vi "xlsx to Cluster.vi"(7 "Excel._SheetName":string="Sheet1", 8 "Error (in)":errorcluster, 11 "file path (dialog if empty)":path) -> (0 "Error (out)":errorcluster, 3 "Parameter Array":T1[](array[typedef]))   [LabVIEW 2020]
uses:
  Controls/Database_Array.ctl
  Controls/Encoding.ctl
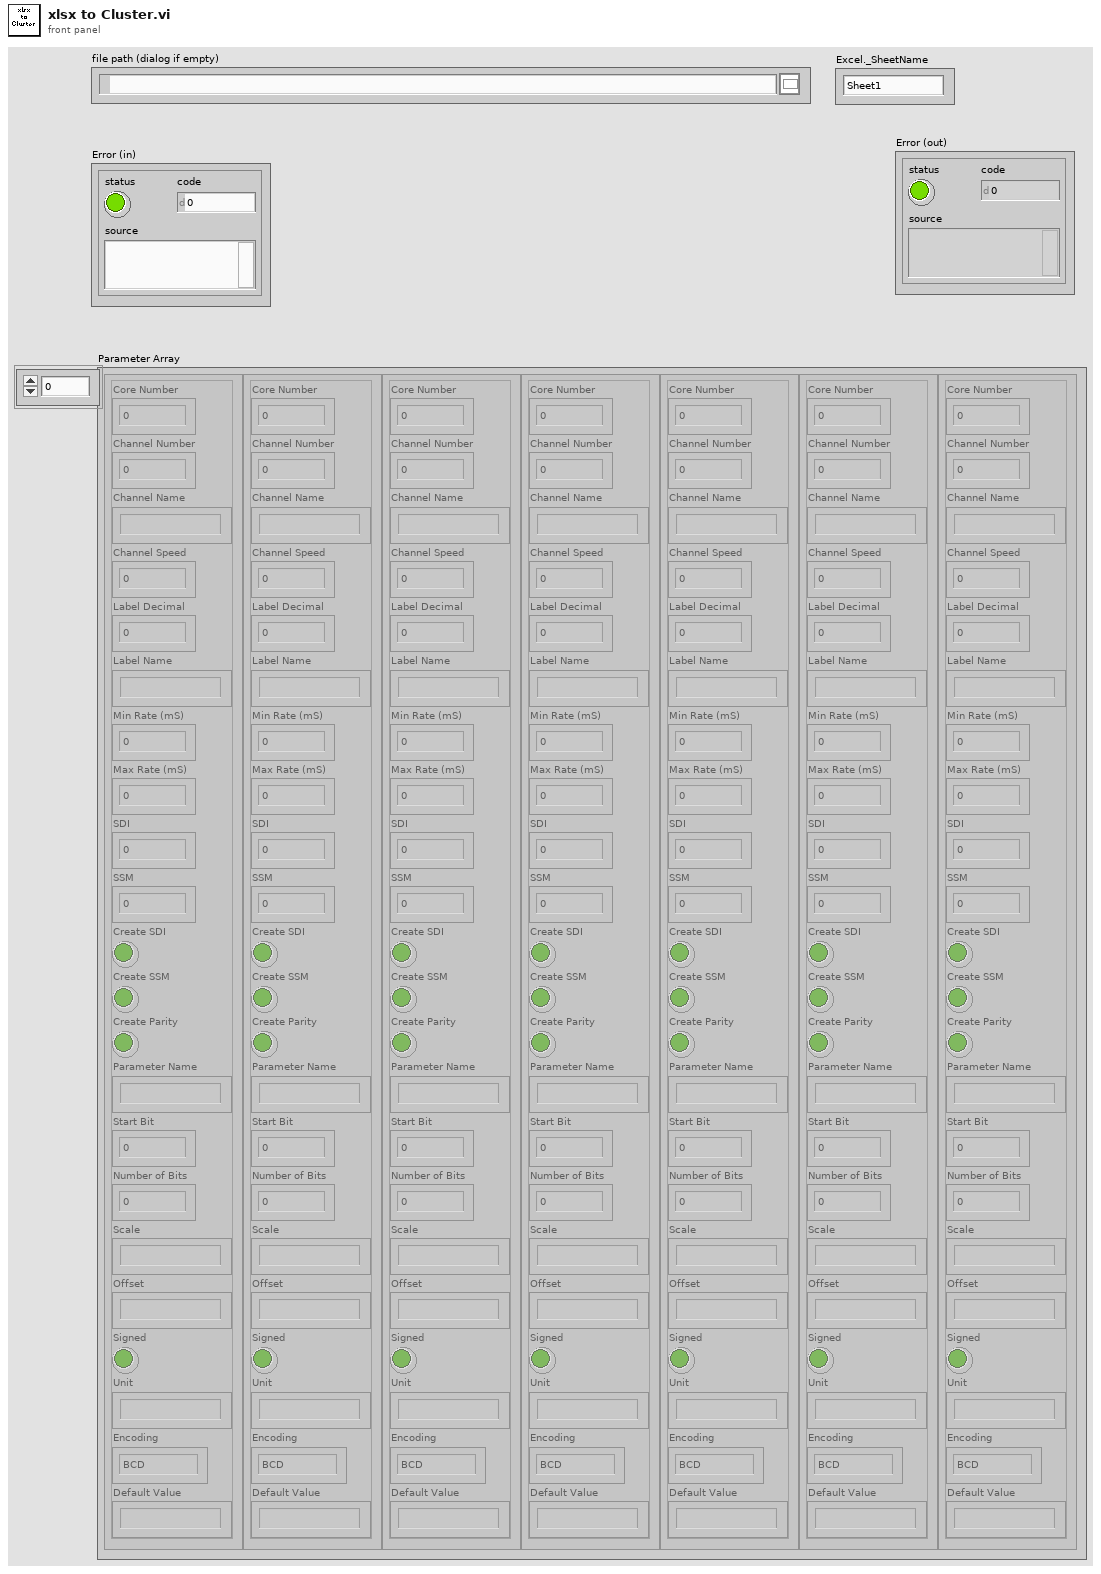
[diagram p1: front panel]
types:
  T1 = typedef "Database_Array.ctl" = cluster{"Core Number":i32, "Channel Number":i32, "Channel Name":string, "Channel Speed":i32, "Label Decimal":i32, "Label Name":string, "Min Rate (mS)":i32, "Max Rate (mS)":i32, "SDI":i32, "SSM":i32, "Create SDI":bool, "Create SSM":bool, "Create Parity":bool, "Parameter Name":string, "Start Bit":i32, "Number of Bits":i32, "Scale":string, "Offset":string, "Signed":bool, "Unit":string, "Encoding":T2, "Default Value":string}
  T2 = typedef "Encoding.ctl" = enum16{"BCD", "BNR", "Discrete"}
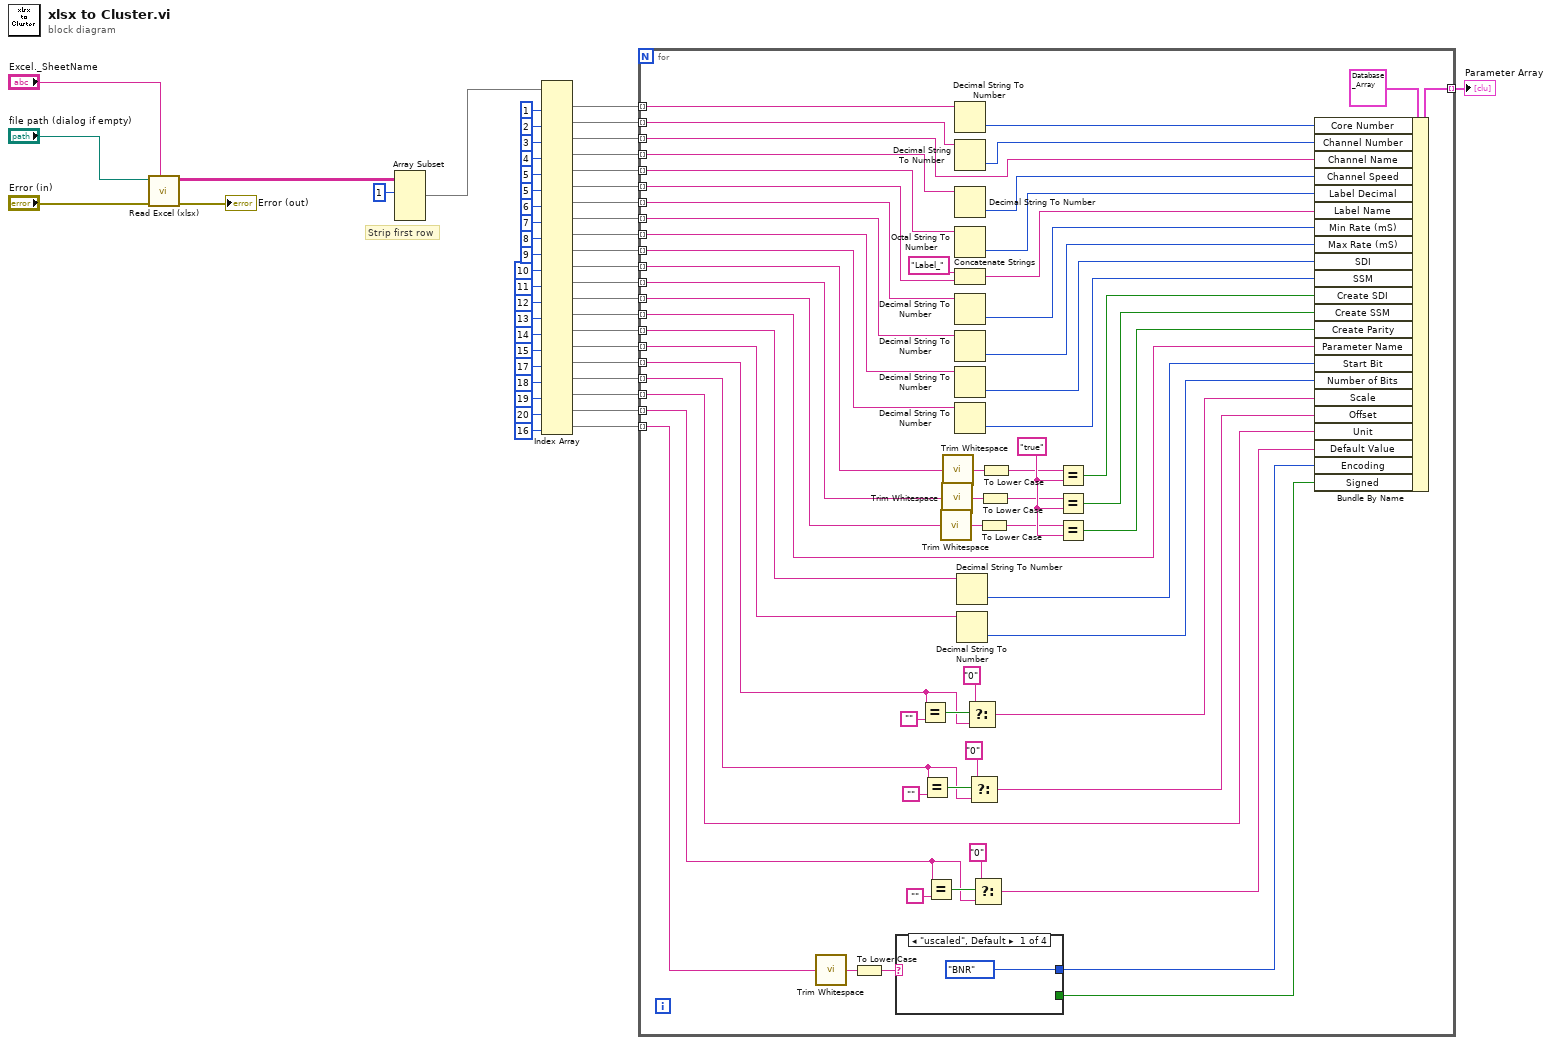
[diagram p0: block diagram]
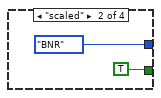
[diagram p2: hidden frame]
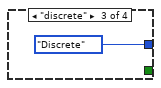
[diagram p3: hidden frame]
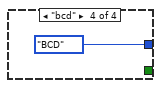
[diagram p4: hidden frame]
diagram:
  # "Strip first row"
  n1 = call "Read Excel (xlsx).vi"("Excel._SheetName"="Excel._SheetName", "error in (no error)"="Error (in)", "File Path Control"="file path (dialog if empty)") -> ("error out"=→"Error (out)":errorcluster, "data"=w48:string[][])  [unwired: 7 in]
  n2 = Array Subset(array=w48, index (row)=1 ("index")) -> (w26:string[][])  [unwired: 3 in]
  n3 = Index Array(array=w26, index (col) #1=1 ("disabled index (col)"), index (col) #2=2 ("disabled index (col)"), index (col) #3=3 ("index (col)"), index (col) #4=4 ("index (col)"), index (col) #5=5 ("index (col)"), index (col) #6=5 ("index (col)"), index (col) #7=6 ("index (col)"), index (col) #8=7 ("index (col)"), index (col) #9=8 ("index (col)"), index (col) #10=9 ("index (col)"), index (col) #11=10 ("index (col)"), index (col) #12=11 ("index (col)"), index (col) #13=12 ("index (col)"), index (col) #14=13 ("index (col)"), index (col) #15=14 ("index (col)"), index (col) #16=15 ("index (col)"), index (col) #17=17 ("index (col)"), index (col) #18=18 ("index (col)"), index (col) #19=19 ("index (col)"), index (col) #20=20 ("index (col)"), index (col) #21=16 ("index (col)")) -> (element #1=w27:string[], element #2=w25:string[], element #3=w24:string[], element #4=w23:string[], element #5=w22:string[], element #6=w21:string[], element #7=w20:string[], element #8=w19:string[], element #9=w18:string[], element #10=w17:string[], element #11=w16:string[], element #12=w15:string[], element #13=w14:string[], element #14=w13:string[], element #15=w12:string[], element #16=w11:string[], element #17=w10:string[], element #18=w9:string[], element #19=w8:string[], element #20=w7:string[], element #21=w6:string[])  [unwired: 21 in]
  n4 = for {
    tunnel: [w110] -> w44 mode=indexing
    tunnel: w27 -> [w108] mode=indexing
    tunnel: w25 -> [w107] mode=indexing
    tunnel: w24 -> [w102] mode=indexing
    tunnel: w23 -> [w105] mode=indexing
    tunnel: w22 -> [w103] mode=indexing
    tunnel: w21 -> [w52] mode=indexing
    tunnel: w20 -> [w101] mode=indexing
    tunnel: w19 -> [w100] mode=indexing
    tunnel: w18 -> [w99] mode=indexing
    tunnel: w17 -> [w98] mode=indexing
    tunnel: w16 -> [w84] mode=indexing
    tunnel: w15 -> [w83] mode=indexing
    tunnel: w14 -> [w81] mode=indexing
    tunnel: w13 -> [w79] mode=indexing
    tunnel: w12 -> [w78] mode=indexing
    tunnel: w11 -> [w77] mode=indexing
    tunnel: w10 -> [w68] mode=indexing
    tunnel: w9 -> [w65] mode=indexing
    tunnel: w8 -> [w64] mode=indexing
    tunnel: w7 -> [w59] mode=indexing
    tunnel: w6 -> [w56] mode=indexing
    w91 = "true"
    n5 = call <vilib>:"Trim Whitespace.vi"("string"=w56) -> ("trimmed string"=w58:string)  [unwired: 1 in]
    n6 = To Lower Case(string=w58) -> (all lower case string=w57:string)
    n7 = case shown="\"uscaled\", Default" w57 {
      tunnel: [Encoding."BNR" ("Enum") Encoding."BNR" ("Enum") Encoding."Discrete" ("Enum") Encoding."BCD" ("Enum")] -> w55
      tunnel: [_ TRUE _ _] -> w54
      frame "uscaled", Default {
      }
      frame "scaled" {
      }
      frame "discrete" {
      }
      frame "bcd" {
      }
    }
    n8 = Equal?(x=w68, y="") -> (x = y?=w73:bool)
    n9 = Equal?(x=w65, y="") -> (x = y?=w70:bool)
    n10 = Equal?(x=w59, y="") -> (x = y?=w62:bool)
    n11 = call <vilib>:"Trim Whitespace.vi"("string"=w81) -> ("trimmed string"=w88:string)  [unwired: 1 in]
    n12 = call <vilib>:"Trim Whitespace.vi"("string"=w83) -> ("trimmed string"=w87:string)  [unwired: 1 in]
    n13 = call <vilib>:"Trim Whitespace.vi"("string"=w84) -> ("trimmed string"=w86:string)  [unwired: 1 in]
    n14 = Decimal String To Number(string=w108) -> (number=w109:i32)  [unwired: 2 in, 1 out]
    n15 = Decimal String To Number(string=w107) -> (number=w106:i32)  [unwired: 2 in, 1 out]
    n16 = Decimal String To Number(string=w105) -> (number=w104:i32)  [unwired: 2 in, 1 out]
    n17 = Octal String To Number(4:w103) -> (0:w96:u32)  [unwired: 2 in, 1 out]
    n18 = Concatenate Strings("Label_" ("String"), w52) -> (w51:string)
    n19 = Decimal String To Number(string=w101) -> (number=w97:i32)  [unwired: 2 in, 1 out]
    n20 = Decimal String To Number(string=w100) -> (number=w95:i32)  [unwired: 2 in, 1 out]
    n21 = Decimal String To Number(string=w99) -> (number=w94:i32)  [unwired: 2 in, 1 out]
    n22 = Decimal String To Number(string=w98) -> (number=w93:i32)  [unwired: 2 in, 1 out]
    n23 = Decimal String To Number(string=w78) -> (number=w76:i32)  [unwired: 2 in, 1 out]
    n24 = Decimal String To Number(string=w77) -> (number=w75:i32)  [unwired: 2 in, 1 out]
    n25 = Select(t="0", s=w73, f=w68) -> (s? t:f=w67:string)
    n26 = Select(t="0", s=w70, f=w65) -> (s? t:f=w66:string)
    n27 = Select(t="0", s=w62, f=w59) -> (s? t:f=w60:string)
    n28 = To Lower Case(string=w88) -> (all lower case string=w80:string)
    n29 = To Lower Case(string=w87) -> (all lower case string=w82:string)
    n30 = To Lower Case(string=w86) -> (all lower case string=w85:string)
    n31 = Equal?(x=w85, y=w91) -> (x = y?=w92:bool)
    n32 = Equal?(x=w82, y=w91) -> (x = y?=w90:bool)
    n33 = Equal?(x=w80, y=w91) -> (x = y?=w89:bool)
    n34 = Bundle By Name(cluster=T1 {"Core Number"=0, "Channel Number"=0, "Channel Name"="", "Channel Speed"=0, "Label Decimal"=0, "Label Name"="", "Min Rate (mS)"=0, "Max Rate (mS)"=0, "SDI"=0, "SSM"=0, "Create SDI"=FALSE, "Create SSM"=FALSE, "Create Parity"=FALSE, "Parameter Name"="", "Start Bit"=0, "Number of Bits"=0, "Scale"="", "Offset"="", "Signed"=FALSE, "Unit"="", "Encoding"=enum."BCD", "Default Value"=""} ("Array"), "Core Number"=w109, "Channel Number"=w106, "Channel Name"=w102, "Channel Speed"=w104, "Label Decimal"=w96, "Label Name"=w51, "Min Rate (mS)"=w97, "Max Rate (mS)"=w95, "SDI"=w94, "SSM"=w93, "Create SDI"=w92, "Create SSM"=w90, "Create Parity"=w89, "Parameter Name"=w79, "Start Bit"=w76, "Number of Bits"=w75, "Scale"=w67, "Offset"=w66, "Unit"=w64, "Default Value"=w60, "Encoding"=w55, "Signed"=w54) -> (w110:T1)
  }
  "Parameter Array" <- w44
